vi "CreateOrganizedLogFolder.vi"(8 "Error In":errorcluster, 10 "Time Stamp":timestamp, 11 "Base Log Path":path) -> (0 "Error Out":errorcluster, 3 "Organized Log Path":path)   [LabVIEW 2013, in "LV-Utilities.lvlib"]
uses:
  LV-Utilities.lvlib
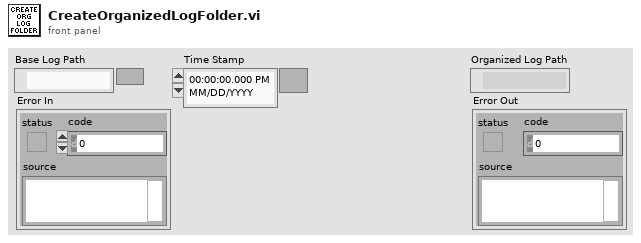
[diagram p1: front panel]
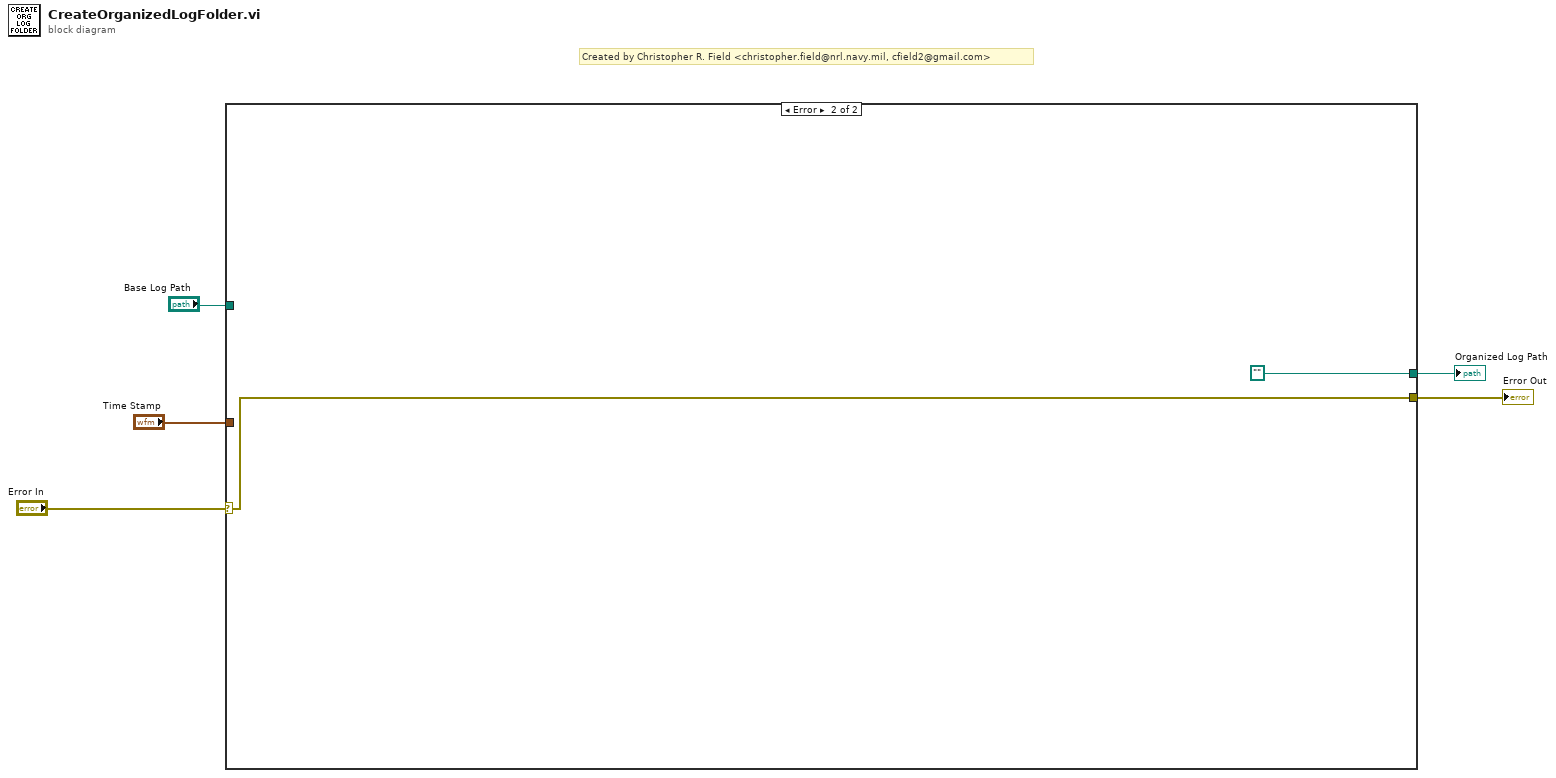
[diagram p0: block diagram]
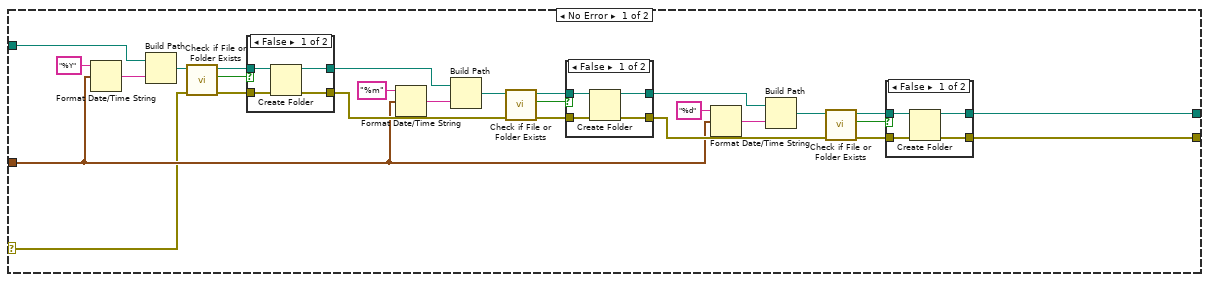
[diagram p2: hidden frame]
diagram:
  # "Created by Christopher R. Field <christopher.field@nrl.navy.mil, cfield2@gmail.com>"
  n1 = case shown="Error" "Error In" {
    selector: "Error In" -> [w6 w52]
    tunnel: "Base Log Path" -> [w26 _]
    tunnel: [w9 path ""] -> w4
    tunnel: [w8 w52] -> w3
    tunnel: "Time Stamp" -> [w7 _]
    frame No Error {
      n2 = Format Date/Time String(time format string (%c)="%Y", seconds (now)=w7) -> (date/time string=w31:string)  [unwired: 1 in]
      n3 = Build Path(base path=w26, name or relative path=w31) -> (appended path=w25:path)
      n4 = call <vilib>:"Check if File or Folder Exists.vi"("error in (no error)"=w6, "path"=w25) -> ("error out"=w22:errorcluster, "file or folder exists?"=w24:bool, "dup path"=w23:path)  [unwired: 7 in]
      n5 = case shown="False" w24 {
        tunnel: w23 -> [w48 w50]
        tunnel: w22 -> [w47 w49]
        tunnel: [w46 w50] -> w21
        tunnel: [w45 w49] -> w19
        frame False {
          n6 = Create Folder(path (use dialog)=w48, error in=w47) -> (created path=w46:path, error out=w45:errorcluster)  [unwired: 1 in, 1 out]
        }
        frame True {
        }
      }
      n7 = Format Date/Time String(time format string (%c)="%m", seconds (now)=w7) -> (date/time string=w29:string)  [unwired: 1 in]
      n8 = Build Path(base path=w21, name or relative path=w29) -> (appended path=w20:path)
      n9 = call <vilib>:"Check if File or Folder Exists.vi"("error in (no error)"=w19, "path"=w20) -> ("error out"=w17:errorcluster, "file or folder exists?"=w16:bool, "dup path"=w18:path)  [unwired: 7 in]
      n10 = case shown="False" w16 {
        tunnel: w18 -> [w42 w44]
        tunnel: w17 -> [w41 w43]
        tunnel: [w40 w44] -> w12
        tunnel: [w39 w43] -> w10
        frame False {
          n11 = Create Folder(path (use dialog)=w42, error in=w41) -> (created path=w40:path, error out=w39:errorcluster)  [unwired: 1 in, 1 out]
        }
        frame True {
        }
      }
      n12 = Format Date/Time String(time format string (%c)="%d", seconds (now)=w7) -> (date/time string=w27:string)  [unwired: 1 in]
      n13 = Build Path(base path=w12, name or relative path=w27) -> (appended path=w11:path)
      n14 = call <vilib>:"Check if File or Folder Exists.vi"("error in (no error)"=w10, "path"=w11) -> ("error out"=w14:errorcluster, "file or folder exists?"=w13:bool, "dup path"=w15:path)  [unwired: 7 in]
      n15 = case shown="False" w13 {
        tunnel: w15 -> [w36 w38]
        tunnel: w14 -> [w35 w37]
        tunnel: [w34 w38] -> w9
        tunnel: [w33 w37] -> w8
        frame False {
          n16 = Create Folder(path (use dialog)=w36, error in=w35) -> (created path=w34:path, error out=w33:errorcluster)  [unwired: 1 in, 1 out]
        }
        frame True {
        }
      }
    }
    frame Error {
    }
  }
  "Organized Log Path" <- w4
  "Error Out" <- w3
